vi "initialize visualizer UI.vi"(5 "Splitter":refnum<vi>, 6 "MCLB Reference":refnum<vi>, 7 "menu reference in":refnum<k9>, 8 "error in (no error)":errorcluster, 9 "display":refnum<vi>, 11 "VI in":refnum<vi>) -> (0 "error out":errorcluster, 2 "selected values":bool[](array[boolean]), 3 "Queue out":refnum<queue>)   [LabVIEW 2016, in "FPGA Resource Manager System Defintion.lvlib"]
uses:
  FPGA Resource Manager System Defintion.lvlib
  viz_command.ctl
  viz_state.ctl
  global constants.vi
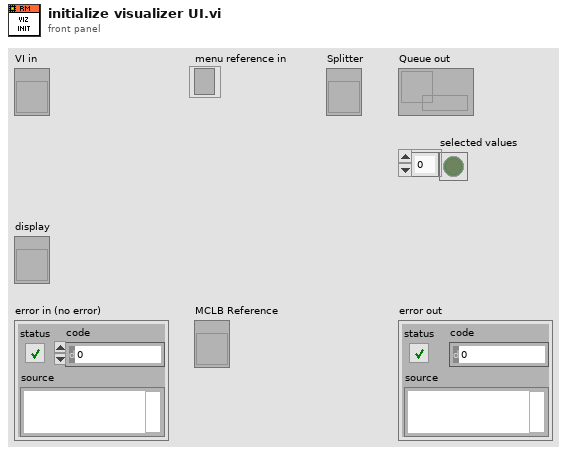
[diagram p1: front panel]
types:
  T1 = enum32{"Invalid", "Standard", "Closed", "Hidden", "Minimized", "Maximized"}
  T2 = typedef "FPGA Resource Manager System Defintion.lvlib/viz_command.ctl" = cluster{"state":T3, "data":variant}
  T3 = typedef "FPGA Resource Manager System Defintion.lvlib/viz_state.ctl" = enum16{"shutdown"}
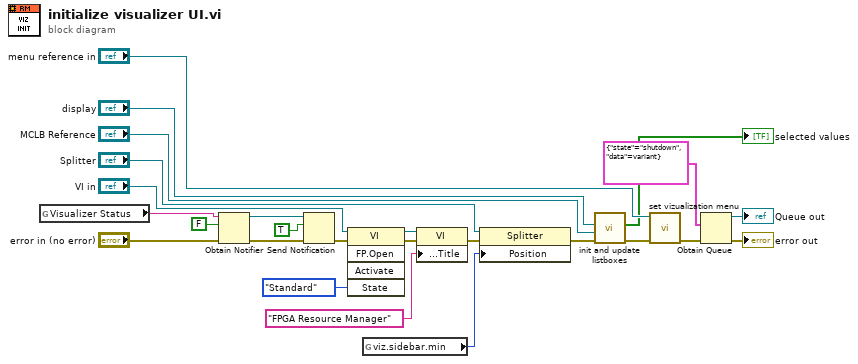
[diagram p0: block diagram]
diagram:
  n1 = global read "global constants.vi" "Visualizer Status"() -> (w21:string)
  n2 = Obtain Notifier(name (unnamed)=w21, notification data type=FALSE, error in (no error)="error in (no error)") -> (notifier out=w19:refnum<notifier>, error out=w17:errorcluster)  [unwired: 1 in, 1 out]
  n3 = Send Notification(notification=TRUE, notifier=w19, error in (no error)=w17) -> (error out=w15:errorcluster)  [unwired: 1 out]
  n4 = invoke class="VI" method="FP.Open"(reference="VI in", error in=w15, "State"=T1."Standard") -> (reference out=w10:refnum<vi>, error out=w24:errorcluster)  [unwired: 2 in, 3 out]
  n5 = global read "global constants.vi" "viz.sidebar.min"() -> (w6:i32)
  n6 = property class="VI"(reference=w10, error in=w24, "Front Panel.Title"="FPGA Resource Manager" ("Front Panel Window:Title")) -> (error out=w8:errorcluster)  [unwired: 1 out]
  n7 = property on="Property Node" class="Splitter"(reference="Splitter", error in=w8, "Position"=w6) -> (error out=w3:errorcluster)  [unwired: 1 out]
  n8 = call "init and update listboxes.vi"("error in (no error)"=w3, "table"="MCLB Reference", "display"="display") -> ("error out"=w2:errorcluster, "selected values"=→"selected values":bool[])  [unwired: 7 in]
  n9 = call "set vizualization menu.vi"("error in (no error)"=w2, "menu reference in"="menu reference in") -> ("error out"=w23:errorcluster)  [unwired: 8 in, 1 out]
  n10 = Obtain Queue(element data type=T2 {"state"=enum."shutdown", "data"=variant} ("viz_command"), error in (no error)=w23) -> (queue out=→"Queue out":refnum<queue>, error out=→"error out":errorcluster)  [unwired: 3 in, 1 out]
